vi "MakeCorrectCommunicationFolder.vi"(0 "Main_dataFolder":path, 3 "SampleName":string) -> (1 "Path Status":string="Path already exist...", 2 "Communication Folder":path)   [LabVIEW 2018]
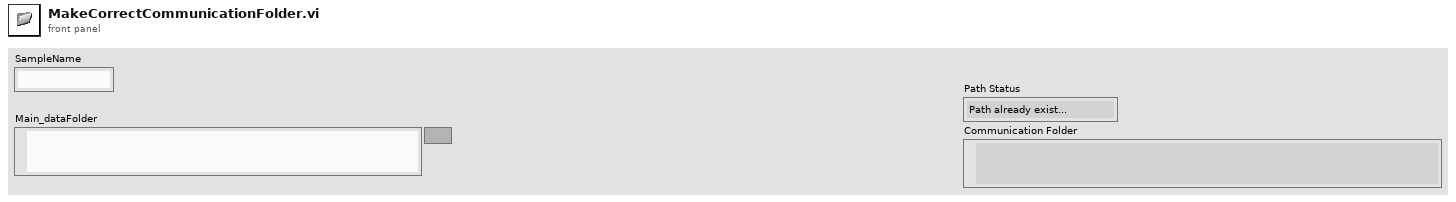
[diagram p1: front panel]
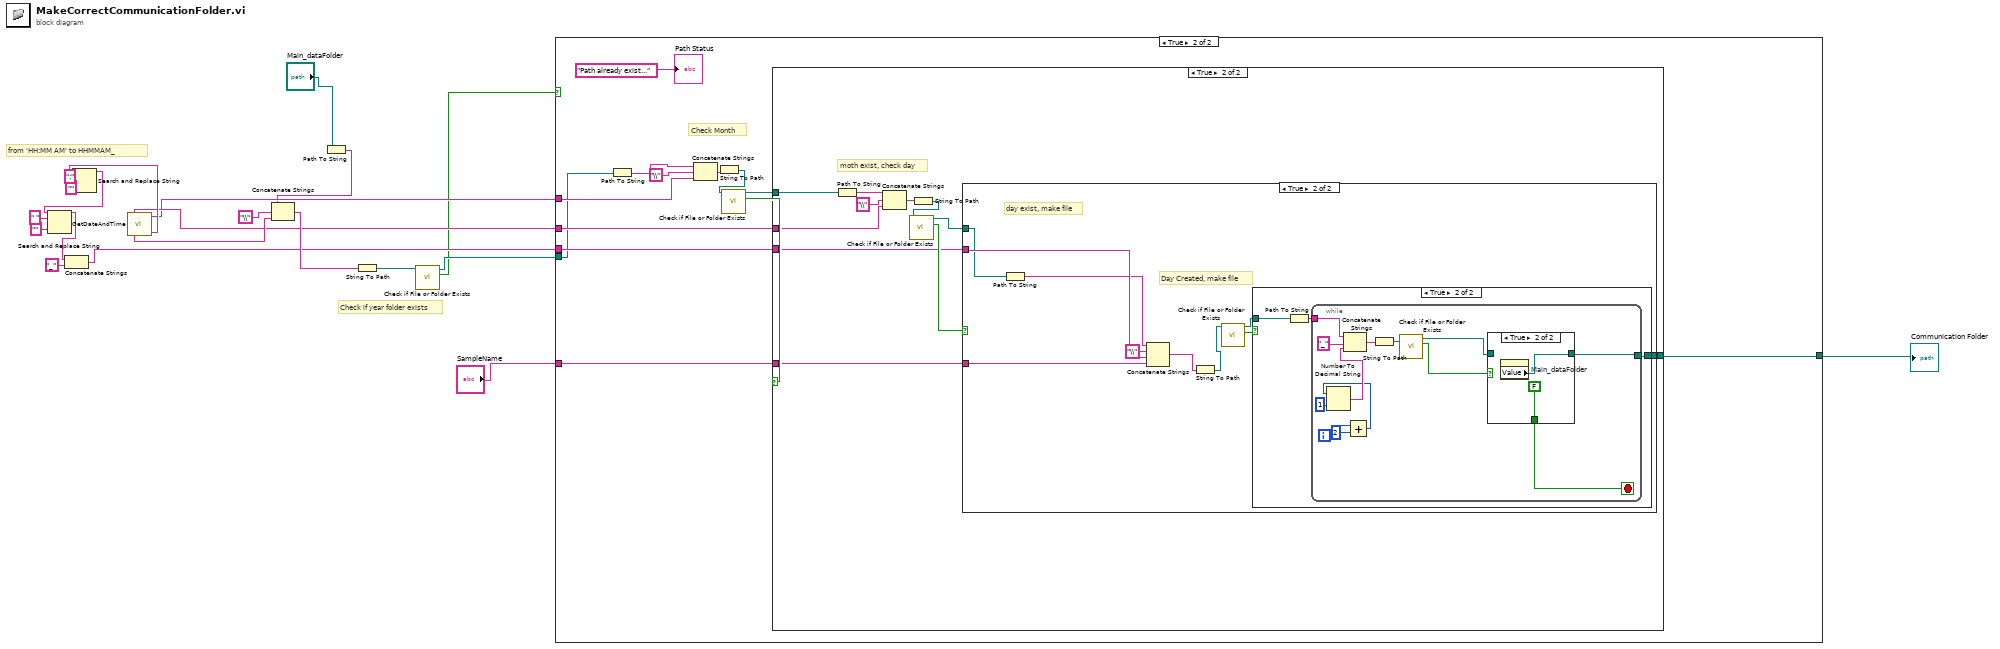
[diagram p0: block diagram]
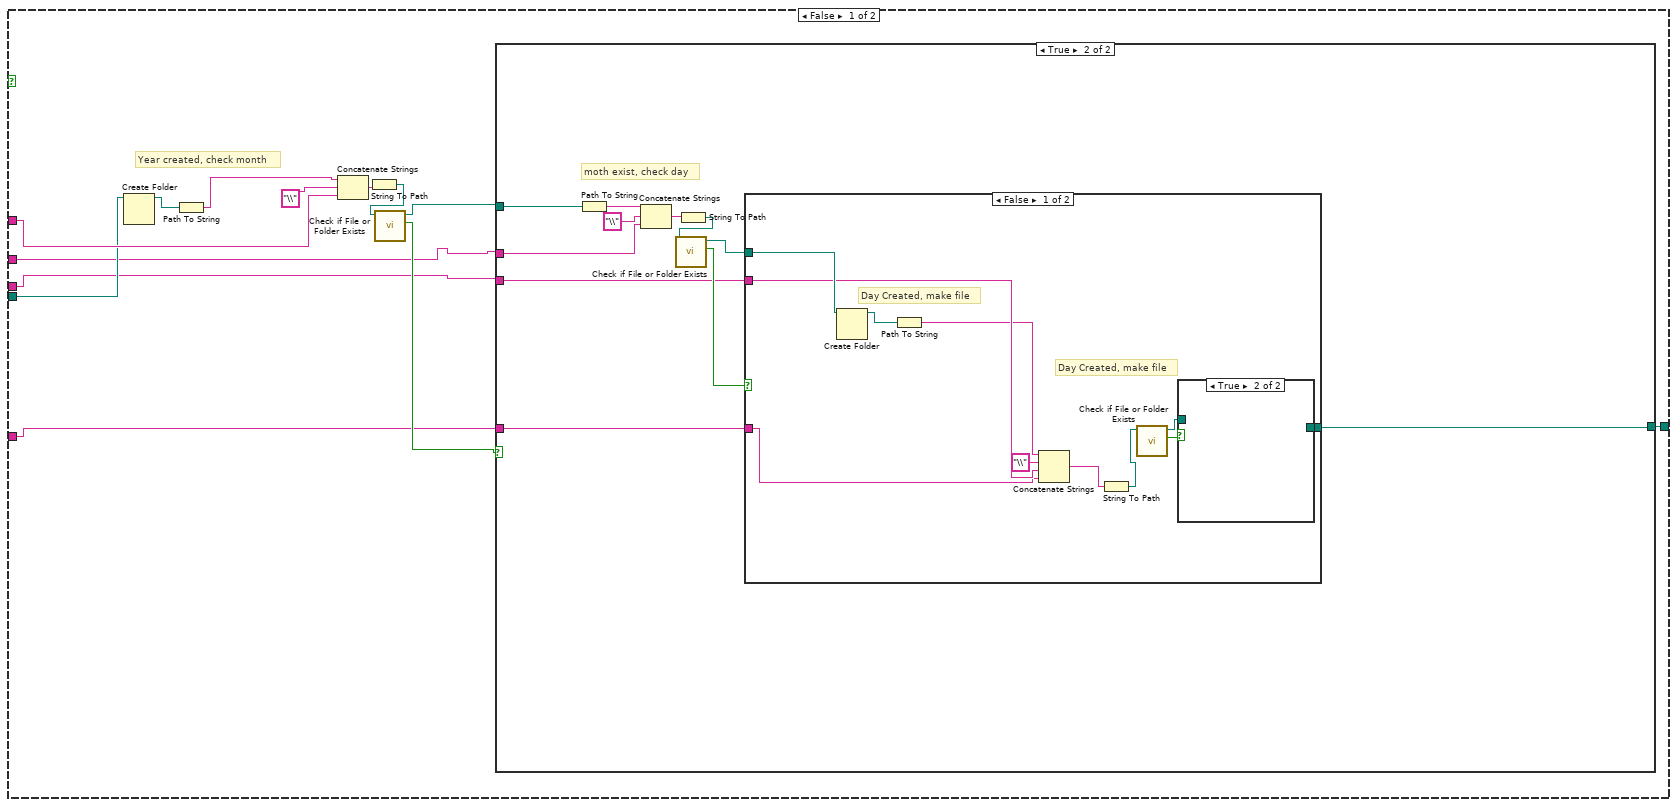
[diagram p2: hidden frame]
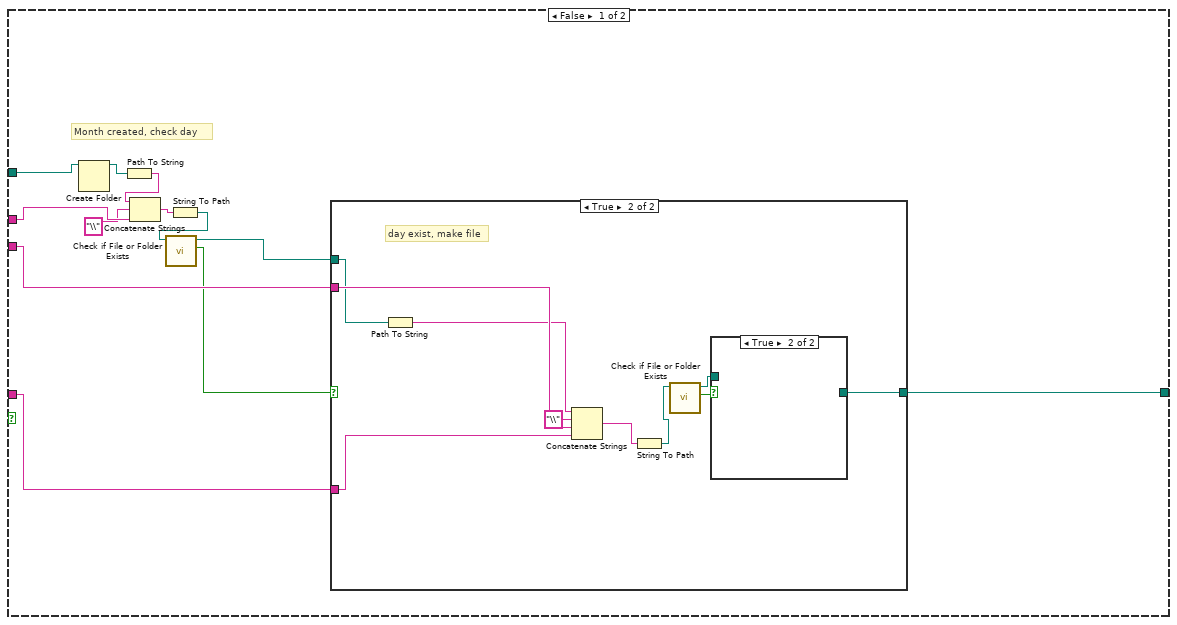
[diagram p3: hidden frame]
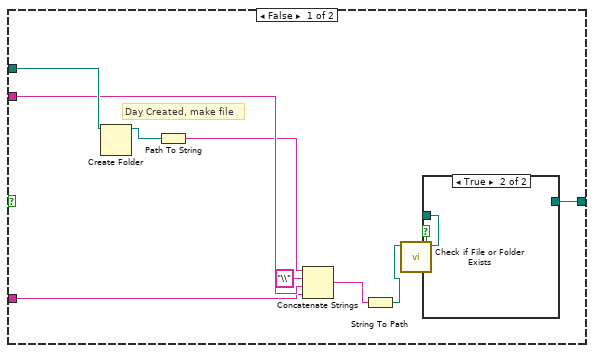
[diagram p4: hidden frame]
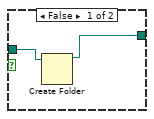
[diagram p5: hidden frame]
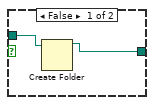
[diagram p6: hidden frame]
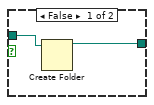
[diagram p7: hidden frame]
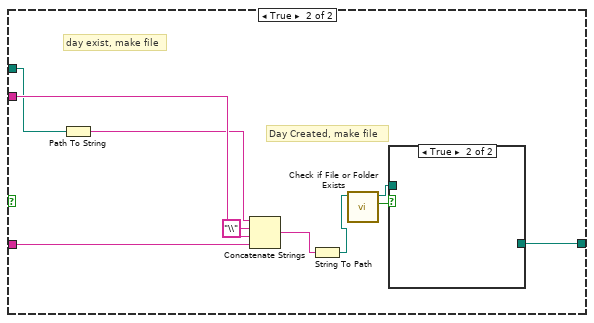
[diagram p8: hidden frame]
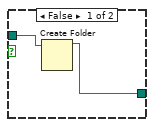
[diagram p9: hidden frame]
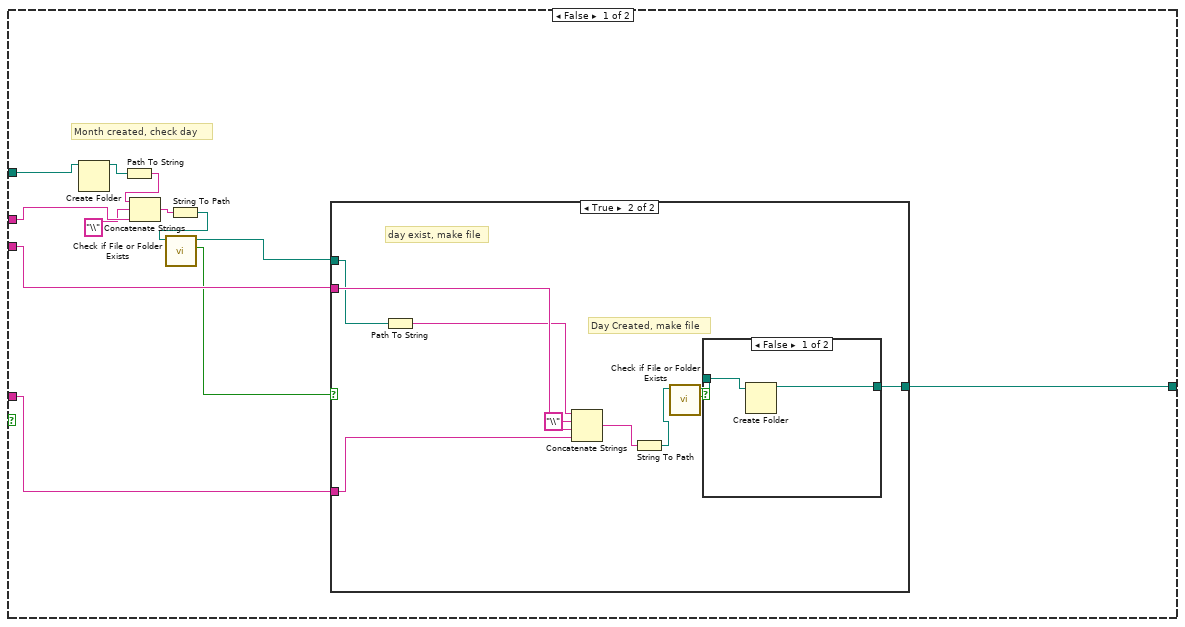
[diagram p10: hidden frame]
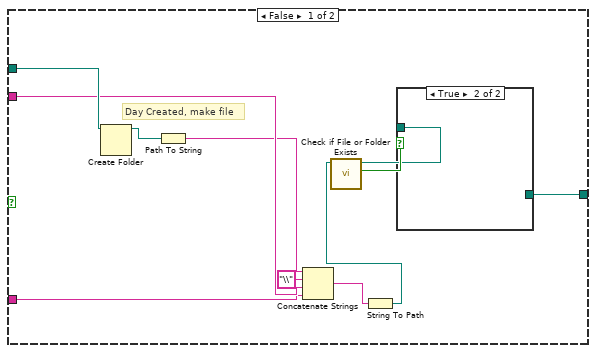
[diagram p11: hidden frame]
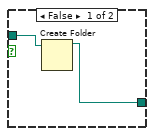
[diagram p12: hidden frame]
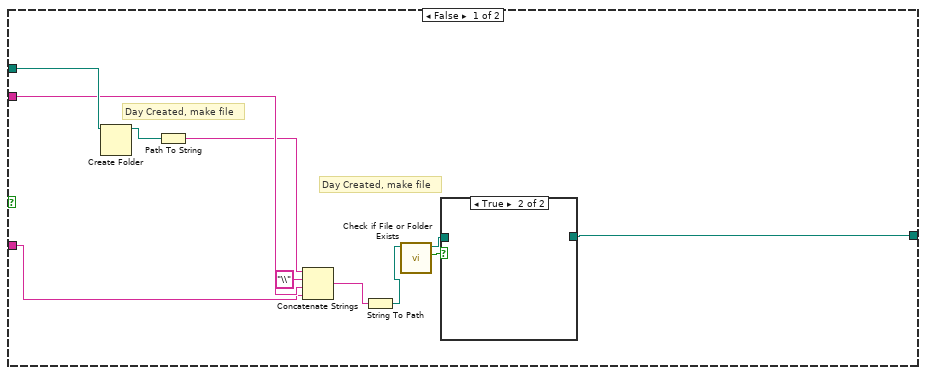
[diagram p14: hidden frame]
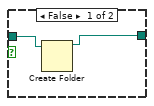
[diagram p15: hidden frame]
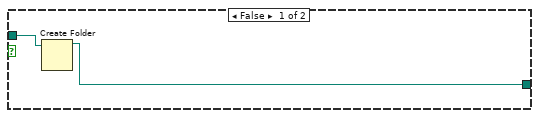
[diagram p16: hidden frame]
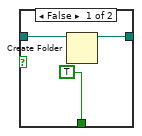
[diagram p17: hidden frame]
diagram:
  # "from 'HH:MM AM' to HHMMAM_"
  # "Check if year folder exists"
  n1 = call "GetDateAndTime.vi"() -> ("Day_clean"=w6:string, "Year_clean"=w18:string, "Month_clean"=w5:string, "time"=w16:string)  [unwired: 1 out]
  n2 = Search and Replace String(input string=w16, search string=":", replace string="" ("replace string (\"\")")) -> (result string=w13:string)  [unwired: 5 in, 3 out]
  n3 = Search and Replace String(input string=w13, search string=" ", replace string="" ("replace string (\"\")")) -> (result string=w12:string)  [unwired: 5 in, 3 out]
  n4 = Concatenate Strings(w12, "_" ("string")) -> (w11:string)
  n5 = Path To String(path="Main_dataFolder") -> (string=w2:string)
  n6 = Concatenate Strings(w2, "\\", w18) -> (w20:string)
  n7 = String To Path(string=w20) -> (path=w19:path)
  n8 = call <vilib>:"Check if File or Folder Exists.vi"("path"=w19) -> ("file or folder exists?"=w3:bool, "dup path"=w17:path)  [unwired: 8 in, 1 out]
  n9 = case shown="True" w3 {
    tunnel: w5 -> [w31 w118]
    tunnel: w6 -> [w23 w113]
    tunnel: w11 -> [w24 w112]
    tunnel: w17 -> [w28 w111]
    tunnel: "SampleName" -> [w25 w109]
    tunnel: [w22 w108] -> w4
    frame False {
      # "Year created, check month"
      n10 = Create Folder(path (use dialog)=w28) -> (created path=w30:path)  [unwired: 2 in, 2 out]
      n11 = Path To String(path=w30) -> (string=w29:string)
      n12 = Concatenate Strings(w29, "\\", w31) -> (w33:string)
      n13 = String To Path(string=w33) -> (path=w32:path)
      n14 = call <vilib>:"Check if File or Folder Exists.vi"("path"=w32) -> ("file or folder exists?"=w26:bool, "dup path"=w27:path)  [unwired: 8 in, 1 out]
      n15 = case shown="True" w26 {
        tunnel: w27 -> [w46 w82]
        tunnel: w23 -> [w45 w79]
        tunnel: w24 -> [w39 w74]
        tunnel: w25 -> [w36 w73]
        tunnel: [w35 w72] -> w22
        frame False {
          # "Month created, check day"
          n16 = Create Folder(path (use dialog)=w46) -> (created path=w43:path)  [unwired: 2 in, 2 out]
          n17 = Path To String(path=w43) -> (string=w42:string)
          n18 = Concatenate Strings(w42, "\\", w45) -> (w41:string)
          n19 = String To Path(string=w41) -> (path=w40:path)
          n20 = call <vilib>:"Check if File or Folder Exists.vi"("path"=w40) -> ("file or folder exists?"=w38:bool, "dup path"=w37:path)  [unwired: 8 in, 1 out]
          n21 = case shown="True" w38 {
            tunnel: w37 -> [w57 w67]
            tunnel: w39 -> [w51 w69]
            tunnel: w36 -> [w48 w61]
            tunnel: [w47 w60] -> w35
            frame False {
              # "Day Created, make file"
              n22 = Create Folder(path (use dialog)=w57) -> (created path=w50:path)  [unwired: 2 in, 2 out]
              n23 = Path To String(path=w50) -> (string=w49:string)
              n24 = Concatenate Strings(w49, "\\" ("string"), w51, w48) -> (w55:string)
              n25 = String To Path(string=w55) -> (path=w54:path)
              n26 = call <vilib>:"Check if File or Folder Exists.vi"("path"=w54) -> ("file or folder exists?"=w53:bool, "dup path"=w52:path)  [unwired: 8 in, 1 out]
              n27 = case shown="True" w53 {
                tunnel: w52 -> [w59 _]
                tunnel: [w58 _] -> w47
                frame False {
                  n28 = Create Folder(path (use dialog)=w59) -> (created path=w58:path)  [unwired: 2 in, 2 out]
                }
                frame True {
                }
              }
            }
            frame True {
              # "day exist, make file"
              n29 = Path To String(path=w67) -> (string=w66:string)
              n30 = Concatenate Strings(w66, "\\" ("string"), w69, w61) -> (w65:string)
              n31 = String To Path(string=w65) -> (path=w64:path)
              n32 = call <vilib>:"Check if File or Folder Exists.vi"("path"=w64) -> ("file or folder exists?"=w63:bool, "dup path"=w62:path)  [unwired: 8 in, 1 out]
              n33 = case shown="True" w63 {
                tunnel: w62 -> [w71 _]
                tunnel: [w70 _] -> w60
                frame False {
                  n34 = Create Folder(path (use dialog)=w71) -> (created path=w70:path)  [unwired: 2 in, 2 out]
                }
                frame True {
                }
              }
            }
          }
        }
        frame True {
          # "moth exist, check day"
          n35 = Path To String(path=w82) -> (string=w81:string)
          n36 = Concatenate Strings(w81, "\\", w79) -> (w78:string)
          n37 = String To Path(string=w78) -> (path=w77:path)
          n38 = call <vilib>:"Check if File or Folder Exists.vi"("path"=w77) -> ("file or folder exists?"=w75:bool, "dup path"=w76:path)  [unwired: 8 in, 1 out]
          n39 = case shown="False" w75 {
            tunnel: w76 -> [w93 w103]
            tunnel: w74 -> [w87 w105]
            tunnel: w73 -> [w84 w97]
            tunnel: [w83 w96] -> w72
            frame False {
              # "Day Created, make file"
              # "Day Created, make file"
              n40 = Create Folder(path (use dialog)=w93) -> (created path=w86:path)  [unwired: 2 in, 2 out]
              n41 = Path To String(path=w86) -> (string=w85:string)
              n42 = Concatenate Strings(w85, "\\" ("string"), w87, w84) -> (w91:string)
              n43 = String To Path(string=w91) -> (path=w90:path)
              n44 = call <vilib>:"Check if File or Folder Exists.vi"("path"=w90) -> ("file or folder exists?"=w89:bool, "dup path"=w88:path)  [unwired: 8 in, 1 out]
              n45 = case shown="True" w89 {
                tunnel: w88 -> [w95 _]
                tunnel: [w94 _] -> w83
                frame False {
                  n46 = Create Folder(path (use dialog)=w95) -> (created path=w94:path)  [unwired: 2 in, 2 out]
                }
                frame True {
                }
              }
            }
            frame True {
              # "Day Created, make file"
              # "day exist, make file"
              n47 = Path To String(path=w103) -> (string=w102:string)
              n48 = Concatenate Strings(w102, "\\" ("string"), w105, w97) -> (w101:string)
              n49 = String To Path(string=w101) -> (path=w100:path)
              n50 = call <vilib>:"Check if File or Folder Exists.vi"("path"=w100) -> ("file or folder exists?"=w99:bool, "dup path"=w98:path)  [unwired: 8 in, 1 out]
              n51 = case shown="True" w99 {
                tunnel: w98 -> [w107 _]
                tunnel: [w106 _] -> w96
                frame False {
                  n52 = Create Folder(path (use dialog)=w107) -> (created path=w106:path)  [unwired: 2 in, 2 out]
                }
                frame True {
                }
              }
            }
          }
        }
      }
    }
    frame True {
      # "Check Month"
      n53 = Path To String(path=w111) -> (string=w110:string)
      n54 = Concatenate Strings(w110, "\\", w118) -> (w117:string)
      n55 = String To Path(string=w117) -> (path=w116:path)
      n56 = call <vilib>:"Check if File or Folder Exists.vi"("path"=w116) -> ("file or folder exists?"=w115:bool, "dup path"=w114:path)  [unwired: 8 in, 1 out]
      n57 = case shown="True" w115 {
        tunnel: w114 -> [w132 w168]
        tunnel: w113 -> [w131 w165]
        tunnel: w112 -> [w125 w160]
        tunnel: w109 -> [w122 w159]
        tunnel: [w121 w158] -> w108
        frame False {
          # "Month created, check day"
          n58 = Create Folder(path (use dialog)=w132) -> (created path=w129:path)  [unwired: 2 in, 2 out]
          n59 = Path To String(path=w129) -> (string=w128:string)
          n60 = Concatenate Strings(w128, "\\", w131) -> (w127:string)
          n61 = String To Path(string=w127) -> (path=w126:path)
          n62 = call <vilib>:"Check if File or Folder Exists.vi"("path"=w126) -> ("file or folder exists?"=w124:bool, "dup path"=w123:path)  [unwired: 8 in, 1 out]
          n63 = case shown="True" w124 {
            tunnel: w123 -> [w143 w153]
            tunnel: w125 -> [w137 w155]
            tunnel: w122 -> [w134 w147]
            tunnel: [w133 w146] -> w121
            frame False {
              # "Day Created, make file"
              n64 = Create Folder(path (use dialog)=w143) -> (created path=w136:path)  [unwired: 2 in, 2 out]
              n65 = Path To String(path=w136) -> (string=w135:string)
              n66 = Concatenate Strings(w135, "\\" ("string"), w137, w134) -> (w141:string)
              n67 = String To Path(string=w141) -> (path=w140:path)
              n68 = call <vilib>:"Check if File or Folder Exists.vi"("path"=w140) -> ("file or folder exists?"=w139:bool, "dup path"=w138:path)  [unwired: 8 in, 1 out]
              n69 = case shown="True" w139 {
                tunnel: w138 -> [w145 _]
                tunnel: [w144 _] -> w133
                frame False {
                  n70 = Create Folder(path (use dialog)=w145) -> (created path=w144:path)  [unwired: 2 in, 2 out]
                }
                frame True {
                }
              }
            }
            frame True {
              # "Day Created, make file"
              # "day exist, make file"
              n71 = Path To String(path=w153) -> (string=w152:string)
              n72 = Concatenate Strings(w152, "\\" ("string"), w155, w147) -> (w151:string)
              n73 = String To Path(string=w151) -> (path=w150:path)
              n74 = call <vilib>:"Check if File or Folder Exists.vi"("path"=w150) -> ("file or folder exists?"=w149:bool, "dup path"=w148:path)  [unwired: 8 in, 1 out]
              n75 = case shown="False" w149 {
                tunnel: w148 -> [w157 _]
                tunnel: [w156 _] -> w146
                frame False {
                  n76 = Create Folder(path (use dialog)=w157) -> (created path=w156:path)  [unwired: 2 in, 2 out]
                }
                frame True {
                }
              }
            }
          }
        }
        frame True {
          # "moth exist, check day"
          n77 = Path To String(path=w168) -> (string=w167:string)
          n78 = Concatenate Strings(w167, "\\", w165) -> (w164:string)
          n79 = String To Path(string=w164) -> (path=w163:path)
          n80 = call <vilib>:"Check if File or Folder Exists.vi"("path"=w163) -> ("file or folder exists?"=w161:bool, "dup path"=w162:path)  [unwired: 8 in, 1 out]
          n81 = case shown="True" w161 {
            tunnel: w162 -> [w179 w189]
            tunnel: w160 -> [w173 w191]
            tunnel: w159 -> [w170 w183]
            tunnel: [w169 w182] -> w158
            frame False {
              # "Day Created, make file"
              # "Day Created, make file"
              n82 = Create Folder(path (use dialog)=w179) -> (created path=w172:path)  [unwired: 2 in, 2 out]
              n83 = Path To String(path=w172) -> (string=w171:string)
              n84 = Concatenate Strings(w171, "\\" ("string"), w173, w170) -> (w177:string)
              n85 = String To Path(string=w177) -> (path=w176:path)
              n86 = call <vilib>:"Check if File or Folder Exists.vi"("path"=w176) -> ("file or folder exists?"=w175:bool, "dup path"=w174:path)  [unwired: 8 in, 1 out]
              n87 = case shown="True" w175 {
                tunnel: w174 -> [w181 _]
                tunnel: [w180 _] -> w169
                frame False {
                  n88 = Create Folder(path (use dialog)=w181) -> (created path=w180:path)  [unwired: 2 in, 2 out]
                }
                frame True {
                }
              }
            }
            frame True {
              # "Day Created, make file"
              # "day exist, make file"
              n89 = Path To String(path=w189) -> (string=w188:string)
              n90 = Concatenate Strings(w188, "\\" ("string"), w191, w183) -> (w187:string)
              n91 = String To Path(string=w187) -> (path=w186:path)
              n92 = call <vilib>:"Check if File or Folder Exists.vi"("path"=w186) -> ("file or folder exists?"=w185:bool, "dup path"=w184:path)  [unwired: 8 in, 1 out]
              n93 = case shown="True" w185 {
                tunnel: w184 -> [w193 w196]
                tunnel: [w192 w194] -> w182
                frame False {
                  n94 = Create Folder(path (use dialog)=w193) -> (created path=w192:path)  [unwired: 2 in, 2 out]
                }
                frame True {
                  n95 = Path To String(path=w196) -> (string=w195:string)
                  n96 = while {
                    tunnel: w195 -> [w209]
                    tunnel: [w202] -> w194
                    i -> [w199]
                    stop <- w205 stop-if-true
                    n97 = Add(x=w199, y=2) -> (x+y=w198:i32)
                    n98 = Number To Decimal String(number=w198, width (-)=i16 1) -> (decimal integer string=w201:string)
                    n99 = Concatenate Strings(w209, "_" ("string"), w201) -> (w207:string)
                    n100 = String To Path(string=w207) -> (path=w204:path)
                    n101 = call <vilib>:"Check if File or Folder Exists.vi"("path"=w204) -> ("file or folder exists?"=w206:bool, "dup path"=w203:path)  [unwired: 8 in, 1 out]
                    n102 = case shown="True" w206 {
                      tunnel: [TRUE FALSE] -> w205
                      tunnel: w203 -> [w211 _]
                      tunnel: [w210 w213] -> w202
                      frame False {
                        n103 = Create Folder(path (use dialog)=w211) -> (created path=w210:path)  [unwired: 2 in, 2 out]
                      }
                      frame True {
                        n104 = property on="Main_dataFolder" class="Path"() -> ("Value"=w213:path)  [unwired: 2 in, 2 out]
                      }
                    }
                  }
                }
              }
            }
          }
        }
      }
      "Path Status" <- "Path already exist..."
    }
  }
  "Communication Folder" <- w4
